vi "Transfer Page.vi"(8 "error in (no error)":errorcluster, 11 "Node Ptr":T1 format="%.0x") -> (0 "error out":errorcluster)   [LabVIEW 2020, in "DSF System Explorer.lvlib"]
uses:
  DSF System Explorer.lvlib
  <vilib>/NI VeriStand/Custom Device API/Custom Device Item Ref.ctl
  DSF Core.lvlibp/Classes/Component User Interface/UI Type.ctl
  <vilib>/NI VeriStand/Custom Device API/Custom Device API.lvlib
  DSF Shared.lvlib
  DSF Core.lvlibp/Classes/Component User Interface/Component User Interfaces.lvclass
  DSF Core.lvlibp/Classes/User Interface/User Interface.lvclass
panel:
  in  "Tab Control":enum32{"Settings"}(tab)
  in  "Header":cluster{"Section Name":string}={"Section Name"="Transfer"}
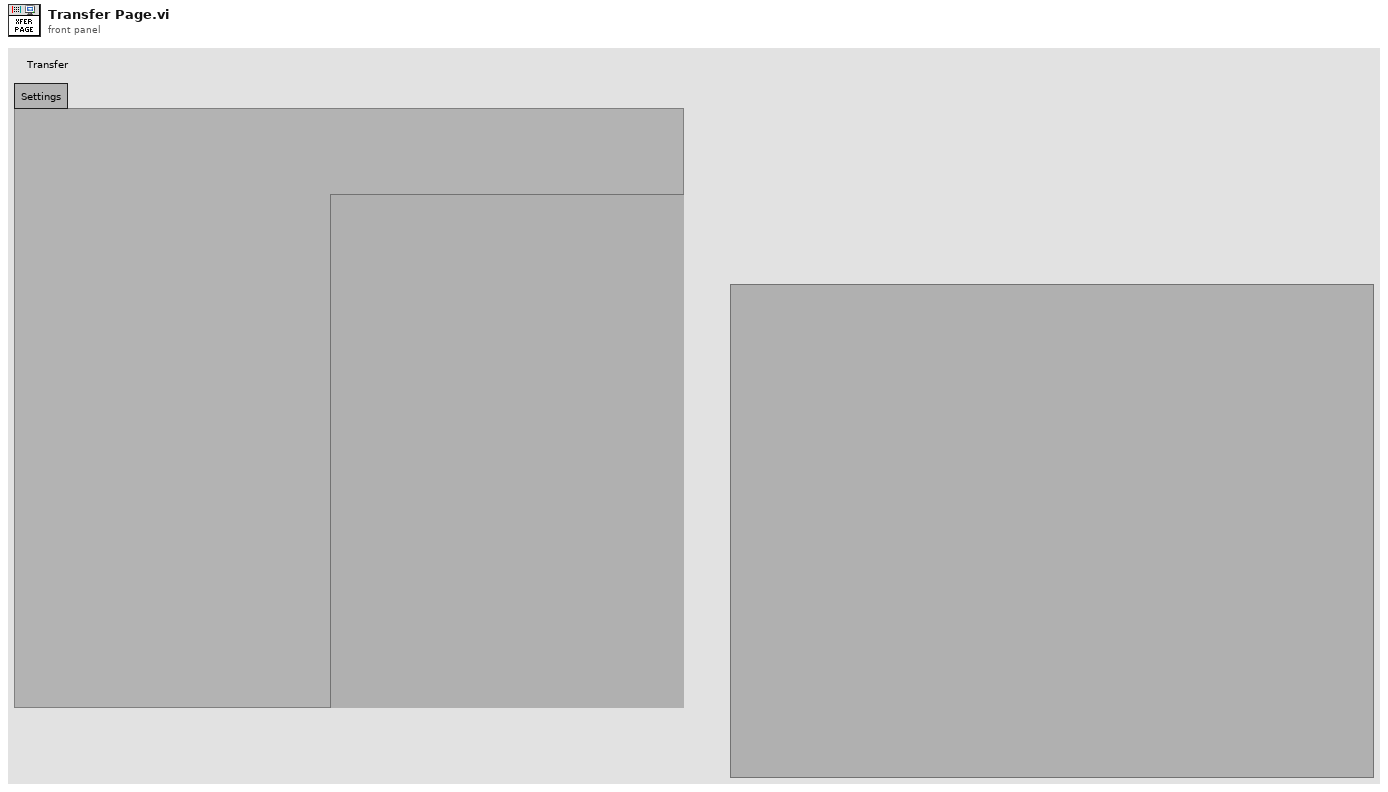
[diagram p1: front panel]
types:
  T1 = typedef "Custom Device API.lvlib/Custom Device Item Ref.ctl" = u64
  T2 = typedef "DSF Core.lvlibp/Component User Interfaces.lvclass/UI Type.ctl" = enum16{"Plugin", "Thread", "Rx Group", "Tx Group", "Rx Transfer", "Tx Transfer", "Rx Channel", "Tx Channel"}
  T3 = typedef "DSF Core.lvlibp/DSF Direction.ctl" = enum8{"Tx", "Rx"}
  T4 = typedef "DSF Core.lvlibp/User Interface Handler.lvclass/User Interface Ref.ctl" = refnum<vi>
  T5 = typedef "DSF Core.lvlibp/DSF Settings Info.ctl" = cluster{"component":string, "values":cluster{"key":string, "value":string}[]}
  T6 = typedef "Custom Device API.lvlib/Custom Device Commands.ctl" = enum16{"Default", "Item renamed", "Shutdown", "Dynamic button pressed"}
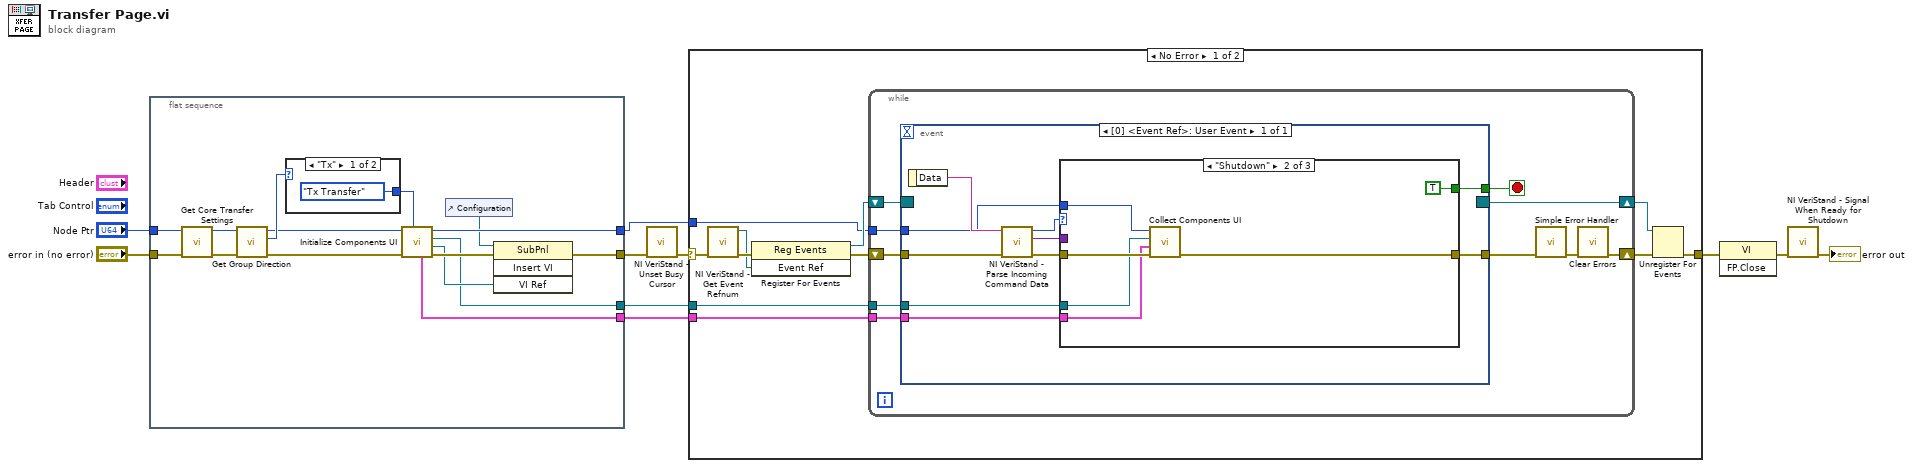
[diagram p0: block diagram]
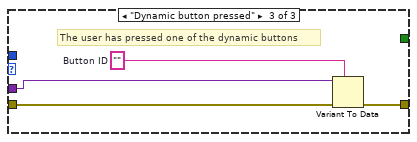
[diagram p3: hidden frame]
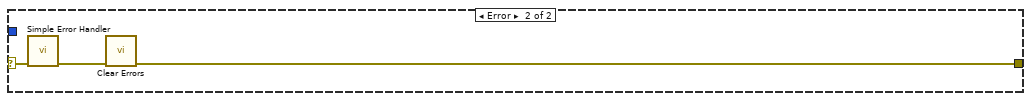
[diagram p4: hidden frame]
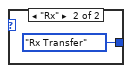
[diagram p5: hidden frame]
diagram:
  n1 = flat-sequence "Initialization code" {
    tunnel: "error in (no error)" -> [w25]
    tunnel: "Node Ptr" -> [w24]
    tunnel: [w17] -> w6
    tunnel: [w13] -> w3
    tunnel: [w14] -> w2
    tunnel: [w11] -> w1
    frame #0 {
      n2 = call "Get Core Transfer Settings.vi"("error in (no error)"=w25, "Item Ref in"=w24) -> ("error out"=w19:errorcluster, "Item Ref out"=w20:T1)  [unwired: 7 in, 1 out]
      n3 = call "Get Group Direction.vi"("error in (no error)"=w19, "Item Ref in"=w20) -> ("error out"=w16:errorcluster, "direction"=w18:T3, "Item Ref out"=w15:T1)  [unwired: 6 in, 1 out]
      n4 = case shown="\"Tx\"" w18 {
        tunnel: [UI_Type."Tx Transfer" ("user interface type") UI_Type."Rx Transfer" ("user interface type")] -> w21
        frame "Tx" {
        }
        frame "Rx" {
        }
      }
      n5 = call "Initialize Components UI.vi"("user interface type"=w21, "error in (no error)"=w16, "Item Ref in"=w15) -> ("error out"=w23:errorcluster, "active vi"=w22:T4, "User Interface Handler"=w14:refnum<class "User Interface Handler.lvclass">, "Item Ref out"=w13:T1, "component settings"=w11:T5[])  [unwired: 4 in]
      n6 = control-ref of="Configuration"() -> (w12:refnum<vi>)
      n7 = invoke class="SubPnl" method="Insert VI"(reference=w12, error in=w23, "VI Ref"=w22) -> (error out=w17:errorcluster)  [unwired: 1 in, 3 out]
    }
  }
  n8 = call <vilib>:"NI VeriStand - Unset Busy Cursor.vi"("error in (no error)"=w6) -> ("error out"=w5:errorcluster)  [unwired: 10 out]
  n9 = case shown="No Error" w5 {
    selector: w5 -> [w30 w72]
    tunnel: [w35 w70] -> w10
    tunnel: w3 -> [w31 _]
    tunnel: w2 -> [w29 _]
    tunnel: w1 -> [w28 _]
    frame No Error {
      n10 = call <vilib>:"NI VeriStand - Get Event Refnum.vi"("error in (no error)"=w30) -> ("error out"=w38:errorcluster, "Event Ref"=w34:refnum<user-event>)  [unwired: 9 out]
      n11 = register-events(error in=w38, w34) -> (reference out=w32:refnum<event-registration>, error out=w33:errorcluster)  [unwired: 1 in]
      n12 = while {
        tunnel: w31 -> [w44]
        shift-right: [w41] -> w36
        shift-left: w33 -> [w47]
        shift-right: [w48] -> w37
        shift-left: w32 -> [w46]
        tunnel: w29 -> [w40]
        tunnel: w28 -> [w39]
        stop <- w45 stop-if-true
        n13 = event shown="[0] <Event Ref>: User Event" {
          selector: w46 -> [_]
          dyn-events: [_] -> w48
          timeout: _ -> [_]
          tunnel: w47 -> [w58]
          tunnel: [w54] -> w45
          tunnel: [w53] -> w43
          tunnel: w44 -> [w52]
          tunnel: w40 -> [w50]
          tunnel: w39 -> [w49]
          event User Event {
            n14 = event-data() -> ("Data"=w57:string)  [unwired: 1 out]
            n15 = call <vilib>:"NI VeriStand - Parse Incoming Command Data.vi"("error in (no error)"=w58, "Incoming data"=w57) -> ("error out"=w56:errorcluster, "Outgoing data"=w51:variant, "Action"=w55:T6)  [unwired: 7 out]
            n16 = case shown="\"Shutdown\"" w55 {
              tunnel: w56 -> [w59 w64 w69]
              tunnel: [_ TRUE _] -> w54
              tunnel: [w59 w63 w66] -> w53
              tunnel: w52 -> [_ w62 _]
              tunnel: w51 -> [_ _ w68]
              tunnel: w50 -> [_ w61 _]
              tunnel: w49 -> [_ w60 _]
              frame "Default", Default {
              }
              frame "Shutdown" {
                n17 = call "Collect Components UI.vi"("error in (no error)"=w64, "current component settings"=w60, "User Interface Handler"=w61, "Item Ref in"=w62) -> ("error out"=w63:errorcluster)  [unwired: 6 in, 1 out]
              }
              frame "Dynamic button pressed" {
                w67 = ""  # Button ID
                # "The user has pressed one of the dynamic buttons"
                n18 = Variant To Data(error in=w69, type=w67, Variant=w68) -> (error out=w66:errorcluster)  [unwired: 1 out]
              }
            }
          }
        }
        n19 = call <vilib>:"Simple Error Handler.vi"("error in (no error)"=w43) -> ("error out"=w42:errorcluster)  [unwired: 1 in, 7 out]
        n20 = call <vilib>:"Clear Errors.vi"("error in (no error)"=w42) -> ("error out"=w41:errorcluster)  [unwired: 1 in, 5 out]
      }
      n21 = Unregister For Events(event registration refnum=w37, error in=w36) -> (error out=w35:errorcluster)
    }
    frame Error {
      n22 = call <vilib>:"Simple Error Handler.vi"("error in (no error)"=w72) -> ("error out"=w71:errorcluster)  [unwired: 1 in, 7 out]
      n23 = call <vilib>:"Clear Errors.vi"("error in (no error)"=w71) -> ("error out"=w70:errorcluster)  [unwired: 1 in, 5 out]
    }
  }
  n24 = invoke class="VI" method="FP.Close"(error in=w10) -> (error out=w9:errorcluster)  [unwired: 2 in, 2 out]
  n25 = call <vilib>:"NI VeriStand - Signal When Ready for Shutdown.vi"("error in (no error)"=w9) -> ("error out"=→"error out":errorcluster)  [unwired: 10 out]
